vi "GetFeaturesForStartupMeas.vi"(8 "error in (no error)":errorcluster, 9 "Metric Cache":variant, 10 "ChannelModel":T9, 11 "DataGroup":T1) -> (0 "error out":errorcluster, 2 "Channels for Startup":T6)   [LabVIEW 2017, in "McsaStartupAnalysis.lvlib"]
uses:
  <vilib>/addons/InsightCM/Devices/Shared/Mcsa/McsaStartupAnalysis/McsaStartupAnalysis.lvlib
  <vilib>/addons/InsightCM/MessageBus/Base/controls/R2_Channel.ctl
  <vilib>/addons/InsightCM/MessageBus/Base/controls/KeyValuePair.ctl
  <vilib>/addons/InsightCM/MessageBus/Base/controls/Metric.ctl
  <vilib>/addons/InsightCM/Devices/Shared/Mcsa/McsaStartupAnalysis/controls/ChannelForStartup.ctl
  <vilib>/addons/InsightCM/Devices/Shared/Mcsa/McsaStartupAnalysis/controls/StartupFeature.ctl
  <vilib>/addons/InsightCM/Devices/Shared/Mcsa/McsaStartupAnalysis/controls/MotorInfo.ctl
  <vilib>/addons/InsightCM/MessageBus/Base/controls/R2_DataGroup.ctl
  <vilib>/addons/InsightCM/MessageBus/Base/controls/OperatingState.ctl
  <vilib>/addons/InsightCM/MessageBus/Base/controls/Trigger.ctl
  <vilib>/addons/InsightCM/MessageBus/Base/controls/Condition.ctl
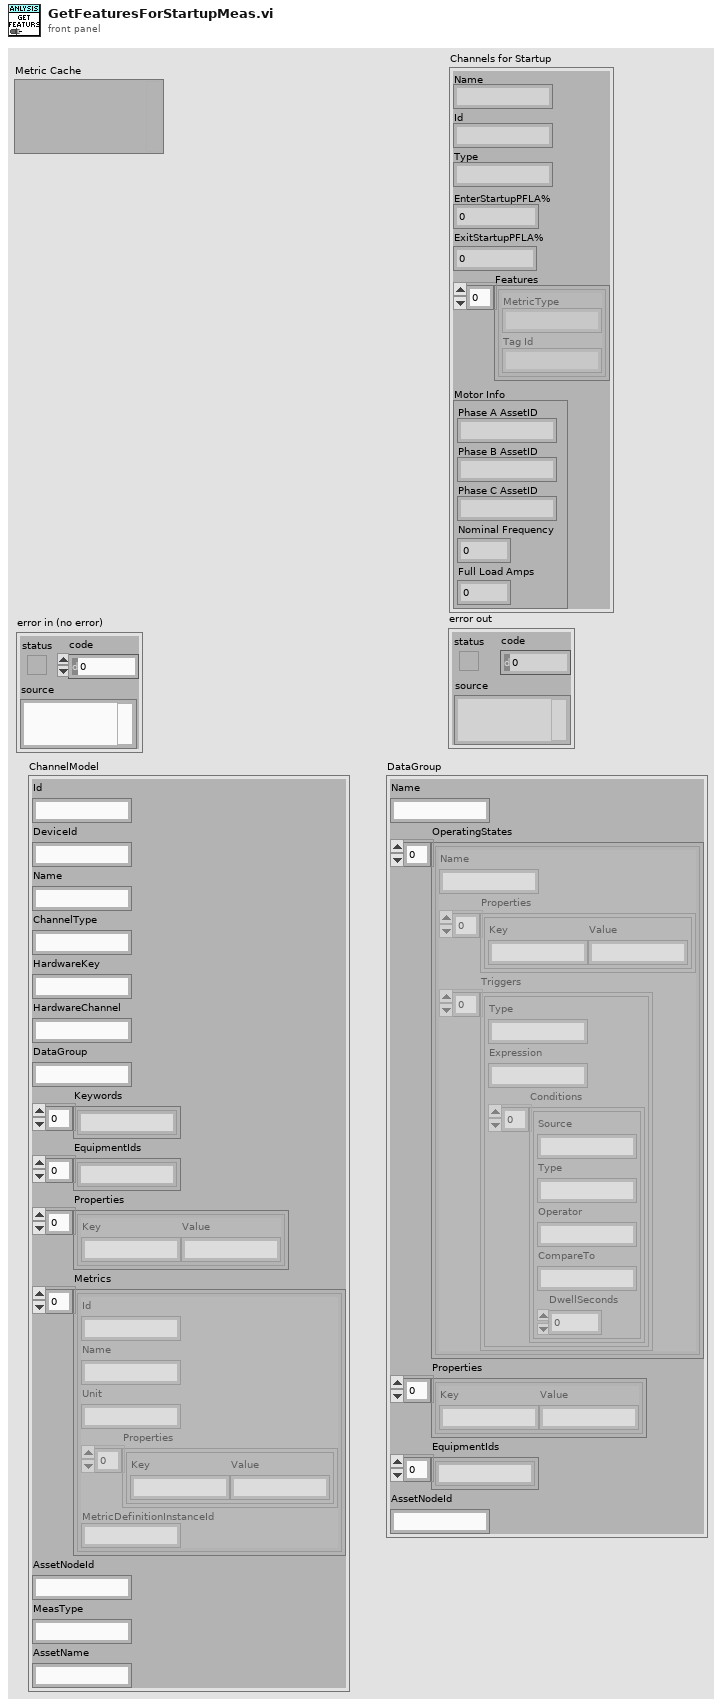
[diagram p1: front panel]
types:
  T1 = typedef "R2_DataGroup.ctl" = cluster{"Name":string, "OperatingStates":T2[], "Properties":T3[], "EquipmentIds":string[], "AssetNodeId":string}
  T2 = typedef "OperatingState.ctl" = cluster{"Name":string, "Properties":T3[], "Triggers":T4[]}
  T3 = typedef "KeyValuePair.ctl" = cluster{"Key":string, "Value":string}
  T4 = typedef "Trigger.ctl" = cluster{"Type":string, "Expression":string, "Conditions":T5[]}
  T5 = typedef "Condition.ctl" = cluster{"Source":string, "Type":string, "Operator":string, "CompareTo":string, "DwellSeconds":dbl}
  T6 = typedef "McsaStartupAnalysis.lvlib/ChannelForStartup.ctl" = cluster{"Name":string, "Id":string, "Type":string, "EnterStartupPFLA%":dbl, "ExitStartupPFLA%":dbl, "Features":T7[], "Motor Info":T8}
  T7 = typedef "McsaStartupAnalysis.lvlib/StartupFeature.ctl" = cluster{"MetricType":string, "Tag Id":string}
  T8 = typedef "McsaStartupAnalysis.lvlib/MotorInfo.ctl" = cluster{"Phase A AssetID":string, "Phase B AssetID":string, "Phase C AssetID":string, "Nominal Frequency":dbl, "Full Load Amps":dbl}
  T9 = typedef "R2_Channel.ctl" = cluster{"Id":string, "DeviceId":string, "Name":string, "ChannelType":string, "HardwareKey":string, "HardwareChannel":string, "DataGroup":string, "Keywords":string[], "EquipmentIds":string[], "Properties":T3[], "Metrics":T10[], "AssetNodeId":string, "MeasType":string, "AssetName":string}
  T10 = typedef "Metric.ctl" = cluster{"Id":string, "Name":string, "Unit":string, "Properties":T3[], "MetricDefinitionInstanceId":string}
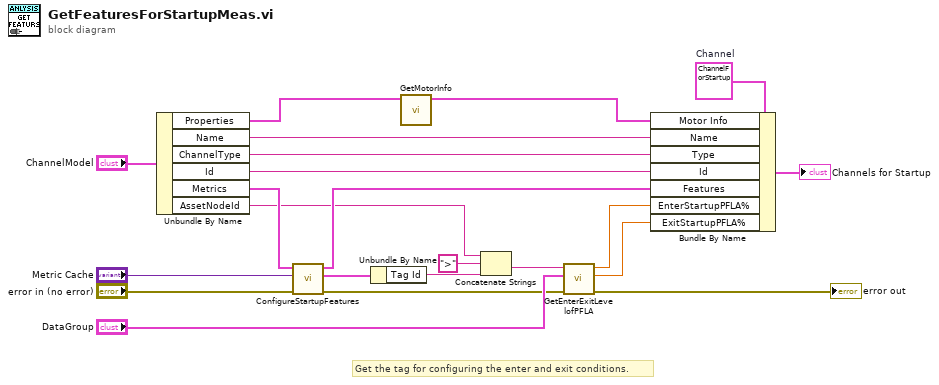
[diagram p0: block diagram]
diagram:
  w16 = T6 {"Name"="", "Id"="", "Type"="", "EnterStartupPFLA%"=0.0, "ExitStartupPFLA%"=0.0, "Features"=[], "Motor Info"={"Phase A AssetID"="", "Phase B AssetID"="", "Phase C AssetID"="", "Nominal Frequency"=0.0, "Full Load Amps"=0.0}}  # Channel
  # "Get the tag for configuring the enter and exit conditions."
  n1 = Unbundle By Name("ChannelModel") -> ("Properties"=w12:T3[], "Name"=w15:string, "ChannelType"=w18:string, "Id"=w19:string, "Metrics"=w2:T10[], "AssetNodeId"=w1:string)
  n2 = call <vilib>:"ConfigureStartupFeatures.vi"("error in (no error)"="error in (no error)", "Metric Cache"="Metric Cache", "Metrics"=w2) -> ("error out"=w4:errorcluster, "PFLA Feature"=w11:T7, "Startup Features"=w20:T7[])  [unwired: 6 in]
  n3 = Unbundle By Name(w11) -> ("Tag Id"=w10:string)
  n4 = call <vilib>:"GetMotorInfo.vi"("Properties"=w12) -> ("Motor Info"=w13:T8)  [unwired: 10 in]
  n5 = Concatenate Strings(w1, ">" ("string"), w10) -> (w8:string)
  n6 = call <vilib>:"GetEnterExitLevelofPFLA.vi"("error in (no error)"=w4, "DataGroup"="DataGroup", "PFLA Source"=w8) -> ("error out"=→"error out":errorcluster, "ExitStartupPFLA%"=w5:dbl, "EnterStartupPFLA%"=w6:dbl)  [unwired: 6 in]
  n7 = Bundle By Name(cluster=w16, "Motor Info"=w13, "Name"=w15, "Type"=w18, "Id"=w19, "Features"=w20, "EnterStartupPFLA%"=w6, "ExitStartupPFLA%"=w5) -> (→"Channels for Startup":T6)
